vi "hamamatsuParameters.vi"() -> ()   [LabVIEW 2017]
panel:
  out "Array 2":T1(array[cluster])
  out "Camera Details Array":T2(array[cluster])
  out "Version Info":T3
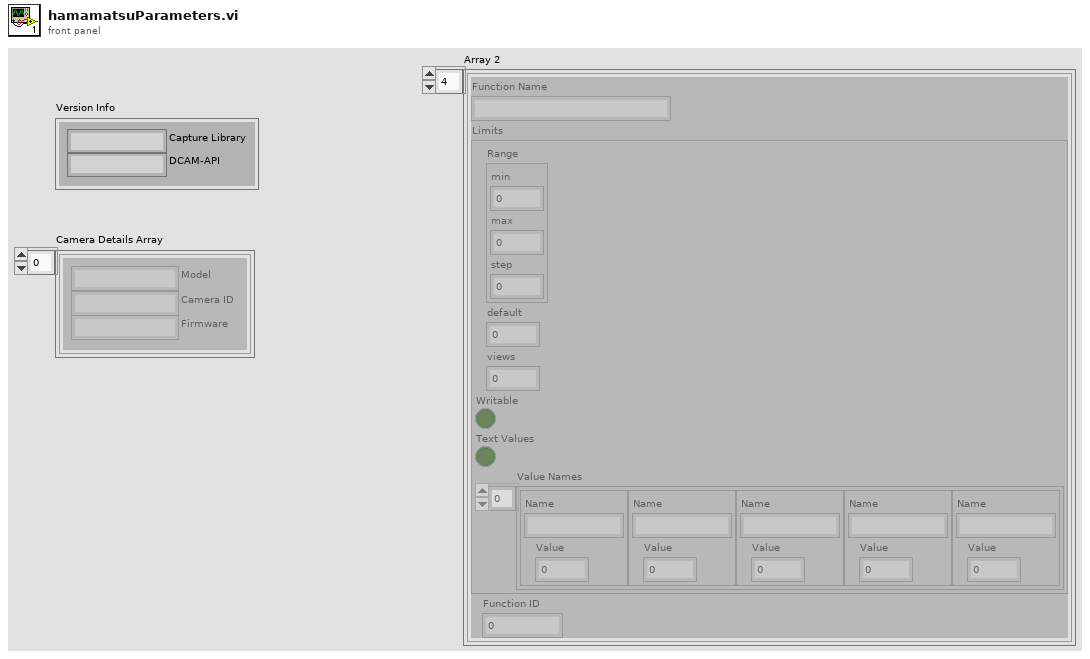
[diagram p1: front panel]
types:
  T1 = cluster{"Function Name":string, "Limits":cluster{"Range":cluster{"min":dbl, "max":dbl, "step":dbl}, "default":dbl, "views":u32, "Writable":bool, "Text Values":bool, "Value Names":cluster{"Name":string, "Value":dbl}[]}, "Function ID":u32}[]
  T2 = cluster{"Model":string, "Camera ID":string, "Firmware":string}[]
  T3 = cluster{"Capture Library":string, "DCAM-API":string}
  T4 = cluster{"Function Name":string, "Function ID":u32}[]
  T5 = cluster{"Range":cluster{"min":dbl, "max":dbl, "step":dbl}, "default":dbl, "views":u32, "Writable":bool, "Text Values":bool, "Value Names":cluster{"Name":string, "Value":dbl}[]}
  T6 = cluster{"Function Name":string, "Limits":cluster{"Range":cluster{"min":dbl, "max":dbl, "step":dbl}, "default":dbl, "views":u32, "Writable":bool, "Text Values":bool, "Value Names":cluster{"Name":string, "Value":dbl}[]}, "Function ID":u32}
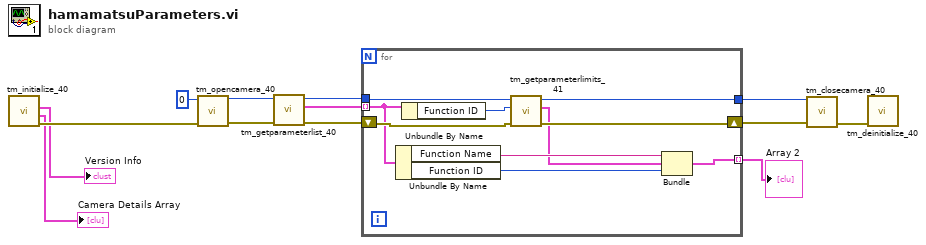
[diagram p0: block diagram]
diagram:
  n1 = call <userlib>:"tm_initialize_40.vi"() -> ("error out"=w12:errorcluster, "Camera Details Array"=→"Camera Details Array":T2, "Version Info"=→"Version Info":T3)  [unwired: 8 in, 1 out]
  n2 = call <userlib>:"tm_opencamera_40.vi"("error in (no error)"=w12, "Camera Index"=u32 0) -> ("error out"=w8:errorcluster, "Handle out"=w9:u32)  [unwired: 7 in, 1 out]
  n3 = call <userlib>:"tm_getparameterlist_40.vi"("error in (no error)"=w8, "Handle in"=w9) -> ("error out"=w6:errorcluster, "Function List"=w7:T4, "Handle out"=w5:u32)  [unwired: 7 in]
  n4 = for {
    tunnel: w5 -> [w23]
    tunnel: w7 -> [w19] mode=indexing
    shift-right: [w20] -> w3
    shift-left: w6 -> [w21]
    tunnel: [w16] -> w1 mode=indexing
    tunnel: [w15] -> w4
    n5 = Unbundle By Name(w19) -> ("Function Name"=w18:string, "Function ID"=w14:u32)
    n6 = Unbundle By Name(w19) -> ("Function ID"=w22:u32)
    n7 = call <userlib>:"tm_getparameterlimits_41.vi"("error in (no error)"=w21, "Parameter"=w22, "Handle in"=w23) -> ("error out"=w20:errorcluster, "Limits"=w17:T5, "Handle out"=w15:u32)  [unwired: 6 in]
    n8 = Bundle("Function Name"=w18, "Limits"=w17, "Function ID"=w14) -> (w16:T6)  [unwired: 1 in]
  }
  "Array 2" <- w1
  n9 = call <userlib>:"tm_closecamera_40.vi"("error in (no error)"=w3, "Handle in"=w4) -> ("error out"=w2:errorcluster)  [unwired: 9 in]
  n10 = call <userlib>:"tm_deinitialize_40.vi"("error in (no error)"=w2) -> ()  [unwired: 10 in, 1 out]
